vi "PRT1_Vi.vi"() -> ()   [LabVIEW 2020]
uses:
  <vilib>/Instr/_visa.llb/VISA Configure Serial Port (Instr).vi
  <vilib>/ptbypt/NI_PtbyPt.lvlib
panel:
  in  "Slide":dbl(slide) scale=-1.0..1.0
  out "VOLTAGE":dbl
  out "BYTE RES":dbl
  in  "SERIAL PORT":refnum<visa-resource-name>
  out "FLUX_GRAPH":dbl(graph)
  out "VOLUME_GRAPH":dbl(graph)
  out "VOLUME [ L ]":dbl
  out "VOLUME_TANK [L]":cluster{dbl, dbl}(slide) scale=0.0..4.0
  out "UPDATED":bool
  out "Respiratoy Rate [bpm]":dbl format="%#_3g"
  out "RESPIRATORY COUNT":dbl
  out "SYSTEM OK":bool
  out "MEAN ERROR":dbl format="%#_4g"
  out "INSPIRATION":bool
  out "SPIRATION":bool
  in  "STOP SYSTEM":bool
  out "PRESSURE CHART":dbl(graph)
  out "FLUX [L/m]":dbl format="%#_4g"
  out "SPEED[cm/s]":dbl format="%#_4g"
  out "PRESSURE":dbl format="%#_4g"
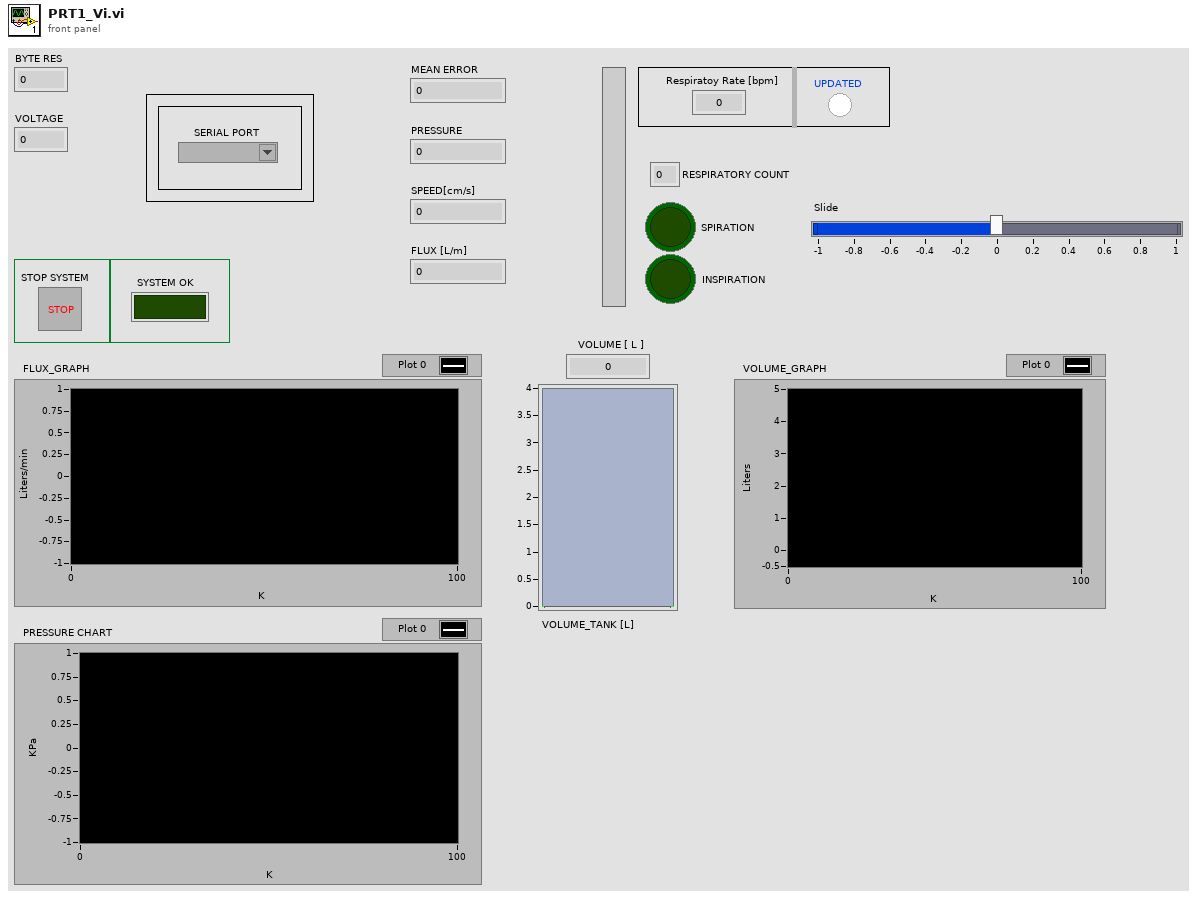
[diagram p1: front panel]
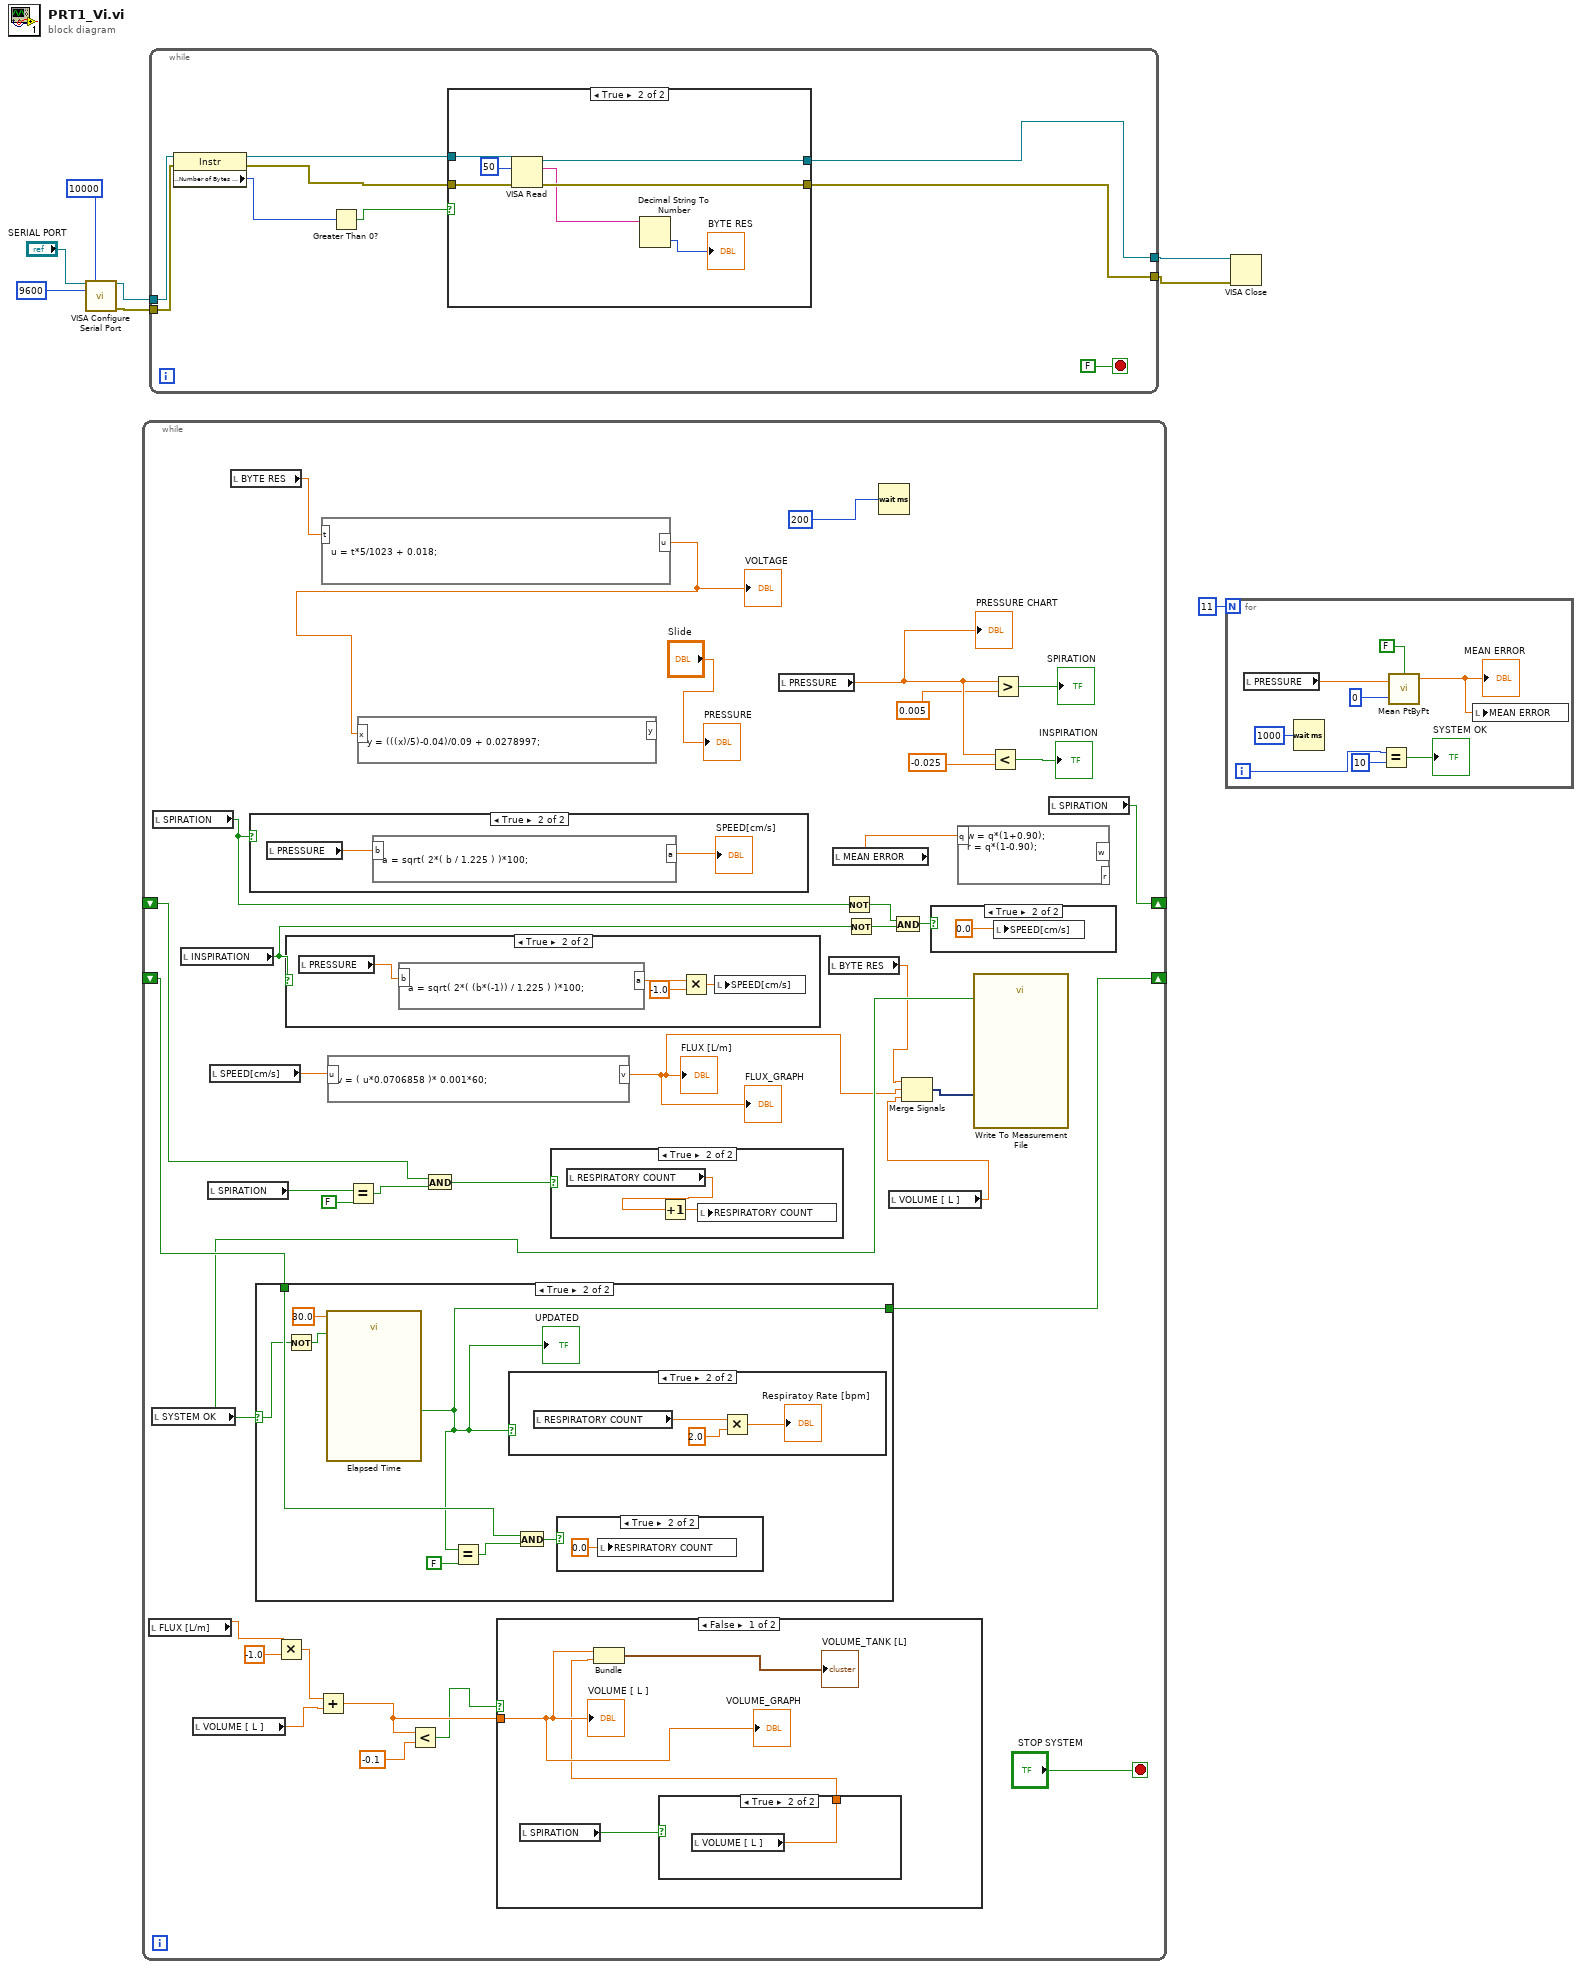
[diagram p0: block diagram]
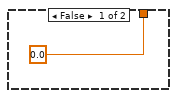
[diagram p3: hidden frame]
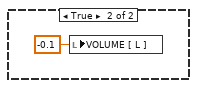
[diagram p4: hidden frame]
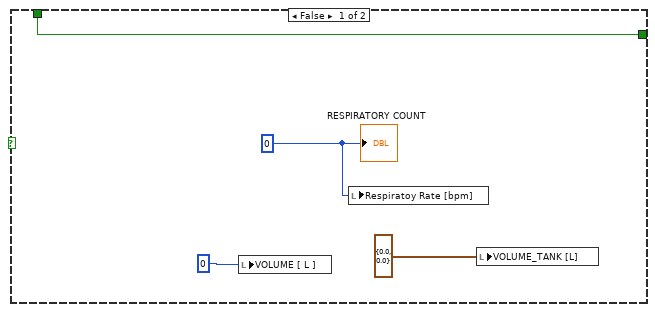
[diagram p8: hidden frame]
diagram:
  n1 = call-poly "VISA Configure Serial Port"("VISA resource name"="SERIAL PORT", "timeout (10sec)"=u32 10000, "baud rate (9600)"=u32 9600) -> ("VISA resource name out"=w5:refnum<visa-resource-name>, "error out"=w4:errorcluster)  [unwired: 11 in]
  n2 = while {
    shift-right: [w42] -> _
    shift-left: _ -> [w41]
    shift-right: [w35] -> _
    shift-left: _ -> [w36]
    stop <- "STOP SYSTEM" stop-if-true
    n3 = local read "FLUX [L/m]"() -> (w23:dbl)
    n4 = local read "SYSTEM OK"() -> (w14:bool)
    n5 = local read "SPIRATION"() -> (w27:bool)
    n6 = local read "INSPIRATION"() -> (w26:bool)
    n7 = local read "VOLUME [ L ]"() -> (w25:dbl)
    n8 = local read "SPIRATION"() -> (w39:bool)
    n9 = local read "SPEED[cm/s]"() -> (w45:dbl)
    n10 = local read "BYTE RES"() -> (w15:dbl)
    n11 = case shown="True" w27 {
      frame False {
      }
      frame True {
        n12 = local read "PRESSURE"() -> (w58:dbl)
        n13 = formula code="a = sqrt( 2*( b / 1.225 ) )*100;"("b"=w58) -> ("a"=→"SPEED[cm/s]":dbl)
      }
    }
    n14 = case shown="True" w14 {
      selector: w14 -> [_ w66]
      tunnel: w36 -> [w62 w68]
      tunnel: [w62 w64] -> w35
      frame False {
        w63 = 0
        n15 = local write "VOLUME [ L ]"(0) -> ()
        n16 = local write "Respiratoy Rate [bpm]"(w63) -> ()
        n17 = local write "VOLUME_TANK [L]"(cluster{dbl, dbl} {0.0, 0.0} ("VOLUME_TANK [L]")) -> ()
        "RESPIRATORY COUNT" <- w63
      }
      frame True {
        n18 = Not(x=w66) -> (.not. x?=w65:bool)
        n19 = call "Elapsed Time"("Time Target (s)"=30.0, "Reset"=w65) -> ("Time has Elapsed"=w64:bool)  [unwired: 10 in, 7 out]
        "UPDATED" <- w64
        n20 = Equal?(x=w64, y=FALSE) -> (x = y?=w70:bool)
        n21 = case shown="True" w64 {
          frame False {
          }
          frame True {
            n22 = local read "RESPIRATORY COUNT"() -> (w74:dbl)
            n23 = Multiply(x=w74, y=2.0) -> (x*y=→"Respiratoy Rate [bpm]":dbl)
          }
        }
        n24 = And(x=w68, y=w70) -> (x .and. y?=w67:bool)
        n25 = case shown="True" w67 {
          frame False {
          }
          frame True {
            n26 = local write "RESPIRATORY COUNT"(0.0 ("RESPIRATORY COUNT")) -> ()
          }
        }
      }
    }
    n27 = Multiply(x=w23, y=-1.0) -> (x*y=w24:dbl)
    n28 = case shown="True" w26 {
      frame False {
      }
      frame True {
        n29 = local read "PRESSURE"() -> (w57:dbl)
        n30 = formula code="a = sqrt( 2*( (b*(-1)) / 1.225 ) )*100;"("b"=w57) -> ("a"=w56:dbl)
        n31 = Multiply(x=w56, y=-1.0) -> (x*y=w54:dbl)
        n32 = local write "SPEED[cm/s]"(w54) -> ()
      }
    }
    n33 = Add(x=w24, y=w25) -> (x+y=w18:dbl)
    n34 = formula code="u = t*5/1023 + 0.018;"("t"=w15) -> ("u"=w20:dbl)
    "VOLTAGE" <- w20
    n35 = formula code="v = ( u*0.0706858 )* 0.001*60;"("u"=w45) -> ("v"=w12:dbl)
    "FLUX [L/m]" <- w12
    "FLUX_GRAPH" <- w12
    n36 = Equal?(x=w39, y=FALSE) -> (x = y?=w40:bool)
    n37 = formula code="y = (((x)/5)-0.04)/0.09 + 0.0278997;"("x"=w20) -> ()  [unwired: 1 out]
    n38 = Less?(x=w18, y=-0.1) -> (x < y?=w16:bool)
    n39 = And(x=w41, y=w40) -> (x .and. y?=w37:bool)
    n40 = case shown="False" w16 {
      tunnel: w18 -> [w48 _]
      frame False {
        n41 = local read "SPIRATION"() -> (w47:bool)
        n42 = case shown="True" w47 {
          tunnel: [0.0 w51] -> w46
          frame False {
          }
          frame True {
            n43 = local read "VOLUME [ L ]"() -> (w51:dbl)
          }
        }
        n44 = Bundle(w48, "VOLUME [ L ]"=w46) -> (→"VOLUME_TANK [L]":cluster{dbl, "VOLUME [ L ]":dbl})  [unwired: 1 in]
        "VOLUME [ L ]" <- w48
        "VOLUME_GRAPH" <- w48
      }
      frame True {
        n45 = local write "VOLUME [ L ]"(-0.1 ("VOLUME [ L ]")) -> ()
      }
    }
    n46 = case shown="True" w37 {
      frame False {
      }
      frame True {
        n47 = local read "RESPIRATORY COUNT"() -> (w77:dbl)
        n48 = Increment(x=w77) -> (x+1=w76:dbl)
        n49 = local write "RESPIRATORY COUNT"(w76) -> ()
      }
    }
    n50 = local read "PRESSURE"() -> (w34:dbl)
    "PRESSURE CHART" <- w34
    n51 = local read "BYTE RES"() -> (w10:dbl)
    n52 = local read "MEAN ERROR"() -> (w33:dbl)
    n53 = Not(x=w27) -> (.not. x?=w29:bool)
    n54 = Not(x=w26) -> (.not. x?=w28:bool)
    n55 = Wait (ms)(milliseconds to wait=u32 200) -> ()  [unwired: 1 out]
    n56 = local read "VOLUME [ L ]"() -> (w11:dbl)
    n57 = And(x=w29, y=w28) -> (x .and. y?=w30:bool)
    n58 = Merge Signals(w10, w12, w11) -> (w9:dynamicdata)
    n59 = case shown="True" w30 {
      frame False {
      }
      frame True {
        n60 = local write "SPEED[cm/s]"(0.0 ("SPEED[cm/s]")) -> ()
      }
    }
    n61 = formula code="w = q*(1+0.90);\nr = q*(1-0.90);"("q"=w33) -> ()  [unwired: 2 out]
    n62 = call "Write To Measurement File"("Signals"=w9, "Enable"=w14) -> ()  [unwired: 15 in, 3 out]
    n63 = Less?(x=w34, y=-0.025) -> (x < y?=→"INSPIRATION":bool)
    n64 = Greater?(x=w34, y=0.005) -> (0:→"SPIRATION":bool)
    n65 = local read "SPIRATION"() -> (w42:bool)
    "PRESSURE" <- "Slide"
  }
  n66 = while {
    tunnel: w5 -> [w83]
    tunnel: w4 -> [w82]
    tunnel: [w78] -> w3
    tunnel: [w81] -> w2
    stop <- FALSE stop-if-true
    n67 = property class="Instr"(reference=w83, error in=w82) -> (reference out=w84:refnum<visa-resource-name>, error out=w85:errorcluster, "Serial Settings:Number of Bytes at Serial Port"=w80:u32)
    n68 = Greater Than 0?(x=w80) -> (x > 0?=w79:bool)
    n69 = case shown="True" w79 {
      tunnel: w85 -> [w87 w95]
      tunnel: w84 -> [w88 w94]
      tunnel: [w88 w93] -> w78
      tunnel: [w87 w92] -> w81
      frame False {
      }
      frame True {
        n70 = VISA Read(VISA resource name=w94, byte count=u32 50, error in (no error)=w95) -> (VISA resource name out=w93:refnum<visa-resource-name>, read buffer=w89:string, error out=w92:errorcluster)  [unwired: 1 out]
        n71 = Decimal String To Number(string=w89) -> (number=→"BYTE RES":i32)  [unwired: 2 in, 1 out]
      }
    }
  }
  n72 = for {
    N: 11 -> [_]
    i -> [w99]
    n73 = local read "PRESSURE"() -> (w102:dbl)
    n74 = Wait (ms)(milliseconds to wait=u32 1000) -> ()  [unwired: 1 out]
    n75 = Equal?(x=w99, y=10) -> (x = y?=→"SYSTEM OK":bool)
    n76 = call <vilib>:"Mean PtByPt.vi"("x"=w102, "sample length"=0, "initialize"=FALSE) -> ("mean"=w96:dbl)  [unwired: 1 in, 1 out]
    "MEAN ERROR" <- w96
    n77 = local write "MEAN ERROR"(w96) -> ()
  }
  n78 = VISA Close(VISA resource name=w3, error in (no error)=w2) -> ()  [unwired: 1 out]
